vi "Finish UI Update.vi"(7 "Main VI":refnum<vi>, 8 "Error In":errorcluster, 11 "State In":T1) -> (0 "Error Out":errorcluster, 3 "State Out":T1)   [LabVIEW 2018, in "Bookmark Manager.lvlib"]
uses:
  Bookmark Manager.lvlib
  Controls/State.ctl
  <vilib>/addons/analyzer/_analyzerctrls.llb/VIAnCtl Analysis App Info.ctl
  Controls/Bookmark.ctl
  Controls/VI Identifier.ctl
  Controls/Bookmarks Groups.ctl
  <vilib>/Utility/miscctls.llb/LVNodeAndColumnTypeDef.ctl
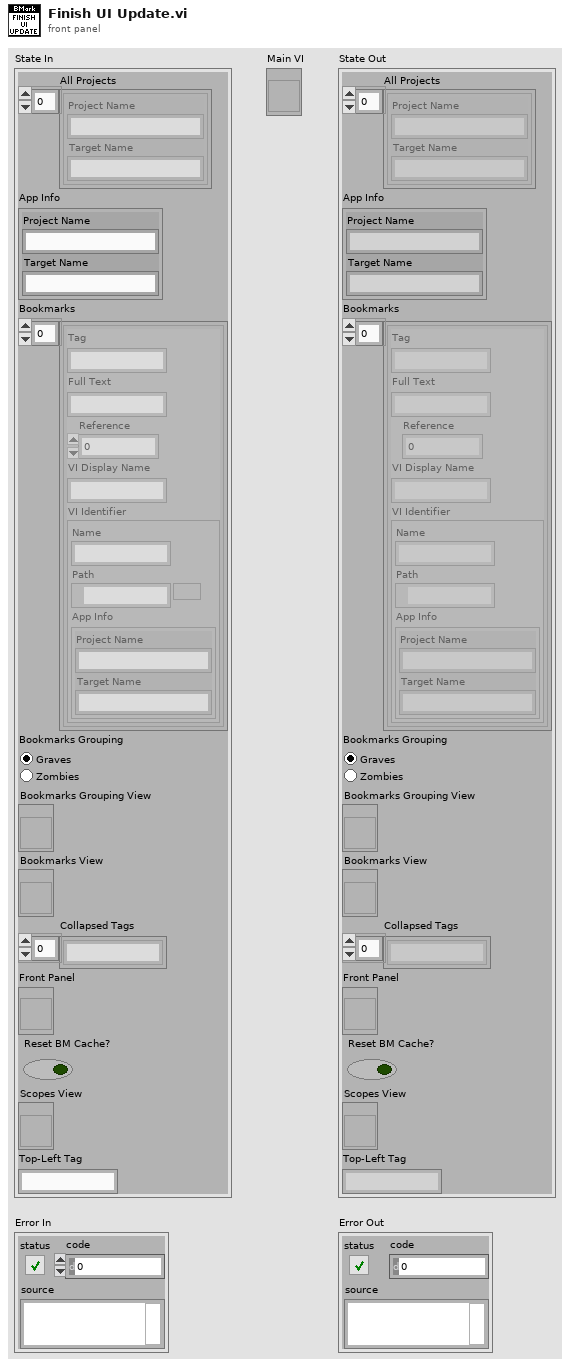
[diagram p1: front panel]
types:
  T1 = typedef "Bookmark Manager.lvlib/State.ctl" = cluster{"All Projects":T2[], "App Info":T2, "Bookmarks":T3[], "Bookmarks Grouping":T5, "Bookmarks Grouping View":refnum<vi>, "Bookmarks View":refnum<vi>, "Collapsed Tags":string[], "Front Panel":refnum<vi>, "Reset BM Cache?":bool, "Scopes View":refnum<vi>, "Top-Left Tag":string}
  T2 = typedef "VIAnCtl Analysis App Info.ctl" = cluster{"Project Name":string, "Target Name":string}
  T3 = typedef "Bookmark Manager.lvlib/Bookmark.ctl" = cluster{"Tag":string, "Full Text":string, "Reference":i32, "VI Display Name":string, "VI Identifier":T4}
  T4 = typedef "Bookmark Manager.lvlib/VI Identifier.ctl" = cluster{"Name":string, "Path":path, "App Info":T2}
  T5 = typedef "Bookmark Manager.lvlib/Bookmarks Groups.ctl" = enum32{"Graves", "Zombies"}
  T6 = typedef "LVNodeAndColumnTypeDef.ctl" = cluster{"Node":string, "Column":i32}
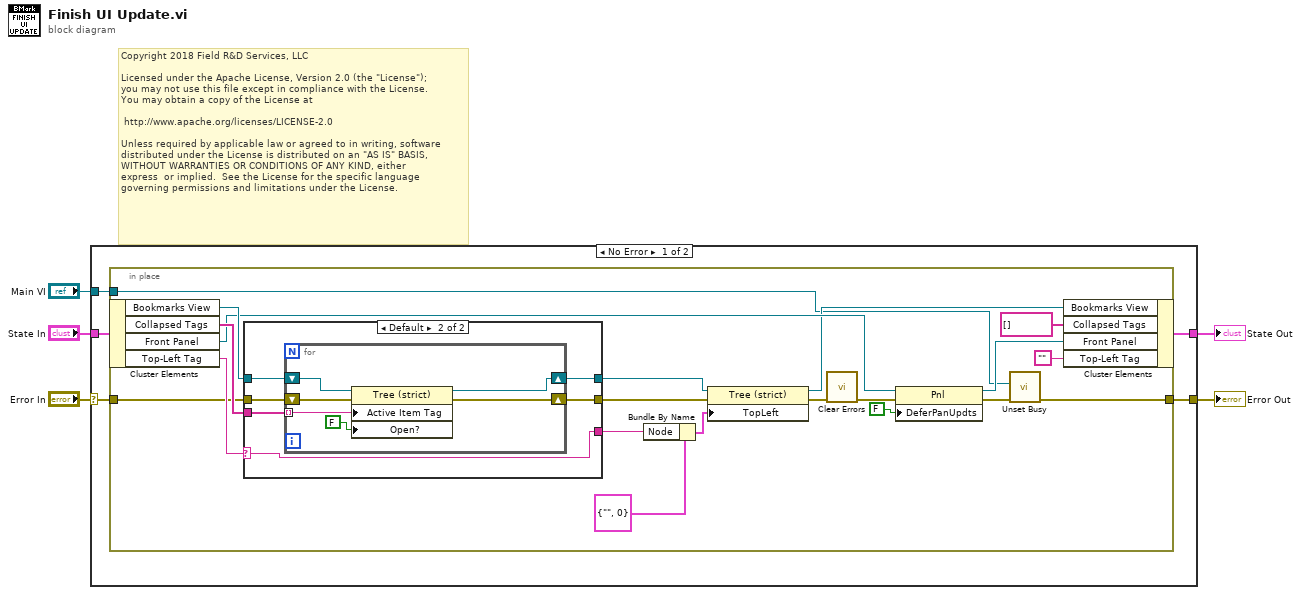
[diagram p0: block diagram]
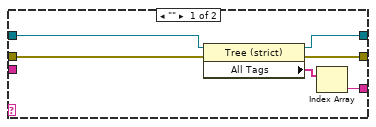
[diagram p2: hidden frame]
diagram:
  # "Copyright 2018 Field R&D Services, LLC\n\nLicensed under the Apache License, Version 2.0 (the \"License\");\nyou may not use this file except in compliance with the License.\nYou may obtain a copy of the License at\n\n\thttp://www.apache.org/licenses/LICENSE-2.0\n\nUnless required by applicable law or agreed to in writing, software\ndistributed under the License is distributed on an \"AS IS\" BASIS,\nWITHOUT WARRANTIES OR CONDITIONS OF ANY KIND, either \nexpress  or implied.  See the License for the specific language \ngoverning permissions and limitations under the License."
  n1 = case shown="No Error" "Error In" {
    selector: "Error In" -> [w7 w49]
    tunnel: [w10 w49] -> w5
    tunnel: [w9 w50] -> w4
    tunnel: "State In" -> [w8 w50]
    tunnel: "Main VI" -> [w6 _]
    frame No Error {
      n2 = in-place {
        in-place-border: w7 -> [w27]
        in-place-border: [w15] -> w10
        in-place-border: w6 -> [w11]
        n3 = in-place-cluster #1(w8) -> ("Bookmarks View"=w28:refnum<vi>, "Collapsed Tags"=w29:string[], "Front Panel"=w20:refnum<vi>, "Top-Left Tag"=w30:string)
        n4 = case shown="Default" w30 {
          selector: w30 -> [_ w42]
          tunnel: w28 -> [w36 w41]
          tunnel: [w35 w40] -> w26
          tunnel: [w33 w42] -> w24
          tunnel: w29 -> [_ w39]
          tunnel: w27 -> [w32 w38]
          tunnel: [w31 w37] -> w25
          frame "" {
            n5 = property class="Tree (strict)"(reference=w36, error in=w32) -> (reference out=w35:refnum<vi>, error out=w31:errorcluster, "All Tags"=w34:string[])
            n6 = Index Array(array=w34) -> (element=w33:string)  [unwired: 1 in]
          }
          frame Default {
            n7 = for {
              shift-right: [w47] -> w40
              shift-left: w41 -> [w48]
              tunnel: w39 -> [w46] mode=indexing
              shift-right: [w43] -> w37
              shift-left: w38 -> [w44]
              n8 = property class="Tree (strict)"(reference=w48, error in=w44, "Active Item Tag"=w46, "Open?"=FALSE) -> (reference out=w47:refnum<vi>, error out=w43:errorcluster)
            }
          }
        }
        n9 = Bundle By Name(cluster=T6 {"Node"="", "Column"=0} ("Top Left Visible Cell"), "Node"=w24) -> (w22:T6)
        n10 = property class="Tree (strict)"(reference=w26, error in=w25, "TopLeft"=w22) -> (reference out=w12:refnum<vi>, error out=w21:errorcluster)
        n11 = call <vilib>:"Clear Errors.vi"("error in (no error)"=w21) -> ("error out"=w18:errorcluster)  [unwired: 5 in, 1 out]
        n12 = property class="Pnl"(reference=w20, error in=w18, "DeferPanUpdts"=FALSE ("Defer Panel Updates")) -> (reference out=w19:refnum<vi>, error out=w16:errorcluster)
        n13 = call <vilib>:"Unset Busy.vi"("error in (no error)"=w16, "VI reference (current VI)"=w11) -> ("error out"=w15:errorcluster)  [unwired: 9 in]
        n14 = in-place-cluster #1("Bookmarks View"=w12, "Collapsed Tags"=string[] [], "Front Panel"=w19, "Top-Left Tag"="") -> (w9:T1)
      }
    }
    frame Error {
    }
  }
  "Error Out" <- w5
  "State Out" <- w4
